vi "Teleop.vi"(10 "Match Info":T1={"Autonomous Elapsed Seconds"=0.0, "TeleOp Elapsed Seconds"=0.0, "Disabled Elapsed Seconds"=0.0, "Visited Autonomous"=FALSE, "Visited TeleOp"=FALSE, "Visited Disabled"=FALSE, "Autonomous Settings"={"Autonomous Style"=enum."Independent", "VI Refnum"=refnum}}, 11 "Call Context":T2) -> ()   [LabVIEW 2012]
doc: "This VI is called for each TeleOp packet received from the DS where the robot is not disabled. It is often used to read from the joysticks and update I/O or to update setpoints for timed control loops. It should complete and return within 20 milliseconds or it may miss DS packets."
uses:
  <vilib>/Rock Robotics/WPI/DriverStation/WPI_DriverStationDerivedRobotMode.ctl
  <vilib>/Rock Robotics/WPI/DriverStation/WPI_DriverStationMatch Info.ctl
  Robot Global Data.vi
  <vilib>/Rock Robotics/WPI/Joystick/WPI_JoystickGetSetRefNum.vi
  State_Machine_Enum.ctl
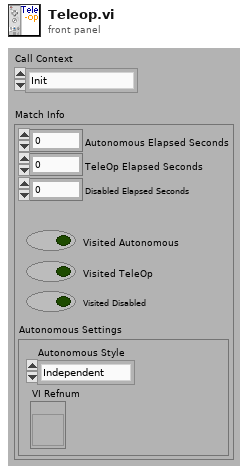
[diagram p1: front panel]
types:
  T1 = typedef "WPI_DriverStationMatch Info.ctl" = cluster{"Autonomous Elapsed Seconds":dbl, "TeleOp Elapsed Seconds":dbl, "Disabled Elapsed Seconds":dbl, "Visited Autonomous":bool, "Visited TeleOp":bool, "Visited Disabled":bool, "Autonomous Settings":cluster{"Autonomous Style":enum16{"Iterative", "Independent"}, "VI Refnum":refnum<vi>}}
  T2 = typedef "WPI_DriverStationDerivedRobotMode.ctl" = enum16{"Init", "Execute", "Stop"}
  T3 = typedef "State_Machine_Enum.ctl" = enum16{"Idle", "Start", "Do", "Stop", "Init"}
  T4 = typedef "WPI_JoystickDevRef.ctl" = cluster{"Device":T5}
  T5 = typedef "WPI_JoystickDeviceEnum.ctl" = enum16{"USB 1", "USB 2", "USB 3", "USB 4", "Kinect 1", "Kinect 2"}
  T6 = typedef "WPI_JoystickButtonState.ctl" = cluster{"Button 1":bool, "Button 2":bool, "Button 3":bool, "Button 4":bool, "Button 5":bool, "Button 6":bool, "Button 7":bool, "Button 8":bool, "Button 9":bool, "Button 10":bool, "Button 11":bool, "Button 12":bool}
  T7 = cluster{"axis 1 (x)":dbl, "axis 2 (y)":dbl, "axis 3 (throttle)":dbl, "axis 4":dbl, "axis 5":dbl, "axis 6":dbl}
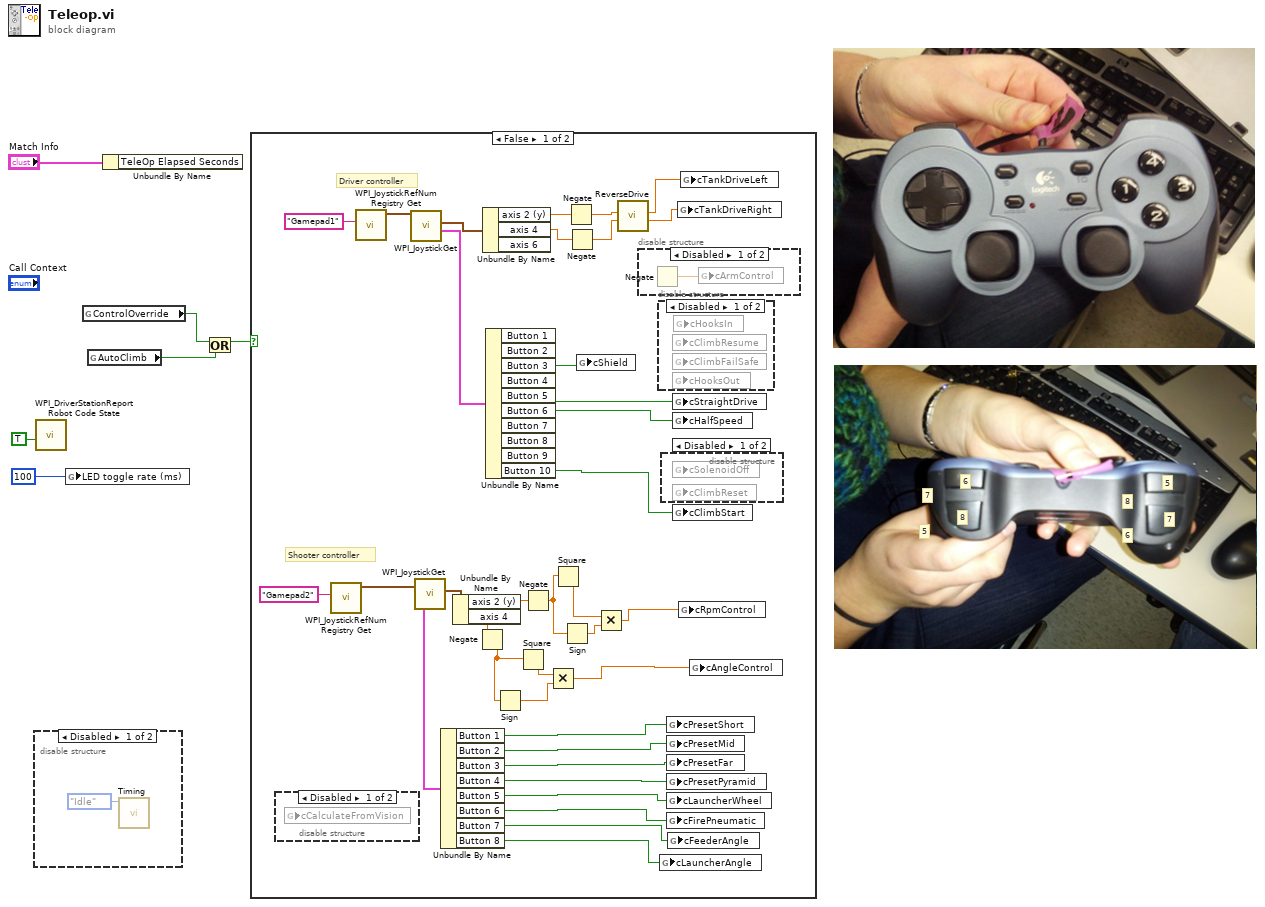
[diagram p0: block diagram]
diagram:
  # "5"
  # "7"
  # "6"
  # "8"
  # "8"
  # "7"
  # "6"
  # "5"
  n1 = disable-structure shown="Disabled" {
    frame Disabled {
      n2 = call "Timing.vi"("State"=State_Machine_Enum."Idle") -> ()  [unwired: 9 in, 2 out]
    }
    frame Enabled {
    }
  }
  n3 = call <vilib>:"WPI_DriverStationReport Robot Code State.vi"("TeleOp"=TRUE ("Autonomous")) -> ()  [unwired: 10 in, 1 out]
  n4 = global write "Robot Global Data.vi" "LED toggle rate (ms)"(u32 100 ("LED ms toggle rate")) -> ()
  n5 = global read "Robot Global Data.vi" "ControlOverride"() -> (w3:bool)
  n6 = global read "Robot Global Data.vi" "AutoClimb"() -> (w1:bool)
  n7 = Unbundle By Name("Match Info") -> ()  [unwired: 1 out]
  n8 = Or(x=w3, y=w1) -> (x .or. y?=w2:bool)
  n9 = case shown="False" w2 {
    frame False {
      # "Shooter controller"
      # "Driver controller"
      n10 = disable-structure shown="Disabled" {
        frame Disabled {
          n11 = global read "Robot Global Data.vi" "cCalculateFromVision"() -> ()  [unwired: 1 in]
        }
        frame Enabled {
        }
      }
      n12 = call <vilib>:"WPI_JoystickRefNum Registry Get.vi"("refnum name"="Gamepad2") -> ("JoystickDevRef"=w41:T4)  [unwired: 1 in, 9 out]
      n13 = call <vilib>:"WPI_JoystickRefNum Registry Get.vi"("refnum name"="Gamepad1") -> ("JoystickDevRef"=w42:T4)  [unwired: 1 in, 9 out]
      n14 = call <vilib>:"WPI_JoystickGet.vi"("JoystickDevRef"=w42) -> ("Buttons"=w37:T6, "Axes"=w39:T7)  [unwired: 4 in, 1 out]
      n15 = call <vilib>:"WPI_JoystickGet.vi"("JoystickDevRef"=w41) -> ("Buttons"=w35:T6, "Axes"=w36:T7)  [unwired: 4 in, 1 out]
      n16 = Unbundle By Name(w35) -> ("Button 1"=w34:bool, "Button 2"=w33:bool, "Button 3"=w32:bool, "Button 4"=w31:bool, "Button 5"=w30:bool, "Button 6"=w29:bool, "Button 7"=w8:bool, "Button 8"=w19:bool)
      n17 = Unbundle By Name(w36) -> ("axis 2 (y)"=w26:dbl, "axis 4"=w24:dbl)
      n18 = Negate(x=w24) -> (-x=w15:dbl)
      n19 = Unbundle By Name(w39) -> ("axis 2 (y)"=w38:dbl, "axis 4"=w12:dbl)  [unwired: 1 out]
      n20 = Unbundle By Name(w37) -> ("Button 3"=w14:bool, "Button 5"=w22:bool, "Button 6"=w20:bool, "Button 10"=w21:bool)  [unwired: 6 out]
      n21 = Sign(1:w15) -> (0:w25:dbl)
      n22 = Square(x=w15) -> (x^2=w23:dbl)
      n23 = Negate(x=w26) -> (-x=w16:dbl)
      n24 = Multiply(x=w23, y=w25) -> (x*y=w17:dbl)
      n25 = Square(x=w16) -> (x^2=w28:dbl)
      n26 = Sign(1:w16) -> (0:w27:dbl)
      n27 = Negate(x=w38) -> (-x=w13:dbl)
      n28 = Negate(x=w12) -> (-x=w11:dbl)
      n29 = global write "Robot Global Data.vi" "cShield"(w14) -> ()
      n30 = Multiply(x=w28, y=w27) -> (x*y=w18:dbl)
      n31 = call "ReverseDrive.vi"("InitLeft"=w13, "InitRight"=w11) -> ("Final Left"=w10:dbl, "FinalRight"=w9:dbl)  [unwired: 7 in]
      n32 = disable-structure shown="Disabled" {
        frame Disabled {
          n33 = Negate() -> (-x=w44:dbl)  [unwired: 1 in]
          n34 = global write "Robot Global Data.vi" "cArmControl"(w44) -> ()
        }
        frame Enabled {
        }
      }
      n35 = disable-structure shown="Disabled" {
        frame Disabled {
          n36 = global read "Robot Global Data.vi" "cClimbResume"() -> ()  [unwired: 1 in]
          n37 = global read "Robot Global Data.vi" "cClimbFailSafe"() -> ()  [unwired: 1 in]
          n38 = global read "Robot Global Data.vi" "cHooksOut"() -> ()  [unwired: 1 in]
          n39 = global read "Robot Global Data.vi" "cHooksIn"() -> ()  [unwired: 1 in]
        }
        frame Enabled {
        }
      }
      n40 = global write "Robot Global Data.vi" "cLauncherAngle"(w19) -> ()
      n41 = disable-structure shown="Disabled" {
        frame Disabled {
          n42 = global read "Robot Global Data.vi" "cSolenoidOff"() -> ()  [unwired: 1 in]
          n43 = global read "Robot Global Data.vi" "cClimbReset"() -> ()  [unwired: 1 in]
        }
        frame Enabled {
        }
      }
      n44 = global write "Robot Global Data.vi" "cPresetShort"(w34) -> ()
      n45 = global write "Robot Global Data.vi" "cPresetMid"(w33) -> ()
      n46 = global write "Robot Global Data.vi" "cPresetFar"(w32) -> ()
      n47 = global write "Robot Global Data.vi" "cPresetPyramid"(w31) -> ()
      n48 = global write "Robot Global Data.vi" "cLauncherWheel"(w30) -> ()
      n49 = global write "Robot Global Data.vi" "cFirePneumatic"(w29) -> ()
      n50 = global write "Robot Global Data.vi" "cFeederAngle"(w8) -> ()
      n51 = global write "Robot Global Data.vi" "cStraightDrive"(w22) -> ()
      n52 = global write "Robot Global Data.vi" "cHalfSpeed"(w20) -> ()
      n53 = global write "Robot Global Data.vi" "cClimbStart"(w21) -> ()
      n54 = global write "Robot Global Data.vi" "cTankDriveRight"(w9) -> ()
      n55 = global write "Robot Global Data.vi" "cRpmControl"(w18) -> ()
      n56 = global write "Robot Global Data.vi" "cTankDriveLeft"(w10) -> ()
      n57 = global write "Robot Global Data.vi" "cAngleControl"(w17) -> ()
    }
    frame True {
    }
  }
